vi "data normalization.vi"() -> ()   [LabVIEW 2025]
panel:
  out "spreadsheet string":string
  out "1D array size":i32
  out "array 2":dbl[](array[numeric])
  out "# of columns":i32
  out "x = y?":bool
  in  "1D worksheet for data processing":string="2.000E+0\t-9.081E-1\t\n2.000E+0\t-9.082E-1\t\n2.000E+0\t-9.083E-1\t\n2.000E+0\t-9.081E-1\t\n2.000E+0\t-9.083E-1\t\n1.750E+0\t-9.075E-1\t\n1.750E+0\t-9.076E-1\t\n1.750E+0\t-9.073E-1\t\n1.750E+0\t-9.075E-1\t\n1.750E+0\t-9.075E-1\t\n1.500E+0\t-9.067E-1\t\n1.500E+0\t-9.068E-1\t\n1.500E+0\t-9.067E-1\t\n1.500E+0\t-9.067E-1\t\n1.500E+0\t-9.067E-1\t\n1.250E+0\t-9.057E-1\t\n1.250E+0\t-9.060E-1\t\n1.250E+0\t-9.059E-1\t\n1.250E+0\t-9.059E-1\t\n1.250E+0\t-9.057E-1\t\n1.000E+0\t-9.109E-1\t\n1.000E+0\t-9.109E-1\t\n1.000E+0\t-9.109E-1\t\n1.000E+0\t-9.108E-1\t\n1.000E+0\t-9.109E-1\t\n7.500E-1\t-9.041E-1\t\n7.500E-1\t-9.042E-1\t\n7.500E-1\t-9.042E-1\t\n7.500E-1\t-9.042E-1\t\n7.500E-1\t-9.042E-1\t\n5.000E-1\t-9.032E-1\t\n5.000E-1\t-9.031E-1\t\n2.000E+0\t-9.086E-1\t\n1.890E+0\t-9.080E-1\t\n1.780E+0\t-9.078E-1\t\n1.670E+0\t-9.074E-1\t\n1.560E+0\t-9.070E-1\t\n1.450E+0\t-9.068E-1\t\n1.340E+0\t-9.121E-1\t\n1.230E+0\t-9.058E-1\t\n1.120E+0\t-9.054E-1\t\n1.010E+0\t-9.111E-1\t\n9.000E-1\t-9.048E-1\t\n7.900E-1\t-9.044E-1\t\n6.800E-1\t-9.038E-1\t\n6.300E-1\t-9.037E-1\t\n5.800E-1\t-9.037E-1\t\n5.300E-1\t-9.033E-1\t\n4.800E-1\t-9.034E-1\t\n4.300E-1\t-9.029E-1\t\n3.800E-1\t-9.029E-1\t\n3.300E-1\t-9.043E-1\t\n2.800E-1\t-9.059E-1\t\n2.300E-1\t-9.135E-1\t\n1.800E-1\t-9.091E-1\t\n1.300E-1\t-9.108E-1\t\n8.000E-2\t-9.123E-1\t\n0.000E+0\t-9.211E-1\t"
  in  "2D Data worksheet":string="2.000E+0\t-9.081E-1\t\n2.000E+0\t-9.082E-1\t\n2.000E+0\t-9.083E-1\t\n2.000E+0\t-9.081E-1\t\n2.000E+0\t-9.083E-1\t\n1.750E+0\t-9.075E-1\t\n1.750E+0\t-9.076E-1\t\n1.750E+0\t-9.073E-1\t\n1.750E+0\t-9.075E-1\t\n1.750E+0\t-9.075E-1\t\n1.500E+0\t-9.067E-1\t\n1.500E+0\t-9.068E-1\t\n1.500E+0\t-9.067E-1\t\n1.500E+0\t-9.067E-1\t\n1.500E+0\t-9.067E-1\t\n1.250E+0\t-9.057E-1\t\n1.250E+0\t-9.060E-1\t\n1.250E+0\t-9.059E-1\t\n1.250E+0\t-9.059E-1\t\n1.250E+0\t-9.057E-1\t\n1.000E+0\t-9.109E-1\t\n1.000E+0\t-9.109E-1\t\n1.000E+0\t-9.109E-1\t\n1.000E+0\t-9.108E-1\t\n1.000E+0\t-9.109E-1\t\n7.500E-1\t-9.041E-1\t\n7.500E-1\t-9.042E-1\t\n7.500E-1\t-9.042E-1\t\n7.500E-1\t-9.042E-1\t\n7.500E-1\t-9.042E-1\t\n5.000E-1\t-9.032E-1\t\n5.000E-1\t-9.031E-1\t\n2.000E+0\t-9.086E-1\t\n1.890E+0\t-9.080E-1\t\n1.780E+0\t-9.078E-1\t\n1.670E+0\t-9.074E-1\t\n1.560E+0\t-9.070E-1\t\n1.450E+0\t-9.068E-1\t\n1.340E+0\t-9.121E-1\t\n1.230E+0\t-9.058E-1\t\n1.120E+0\t-9.054E-1\t\n1.010E+0\t-9.111E-1\t\n9.000E-1\t-9.048E-1\t\n7.900E-1\t-9.044E-1\t\n6.800E-1\t-9.038E-1\t\n6.300E-1\t-9.037E-1\t\n5.800E-1\t-9.037E-1\t\n5.300E-1\t-9.033E-1\t\n4.800E-1\t-9.034E-1\t\n4.300E-1\t-9.029E-1\t\n3.800E-1\t-9.029E-1\t\n3.300E-1\t-9.043E-1\t\n2.800E-1\t-9.059E-1\t\n2.300E-1\t-9.135E-1\t\n1.800E-1\t-9.091E-1\t\n1.300E-1\t-9.108E-1\t\n8.000E-2\t-9.123E-1\t\n0.000E+0\t-9.211E-1\t"
  # "Modify the diagram inside the For Loop"
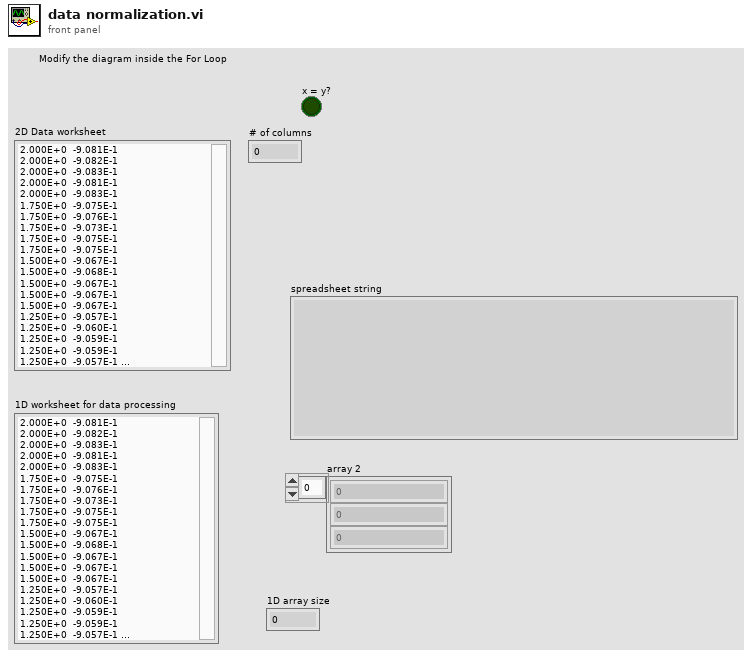
[diagram p1: front panel]
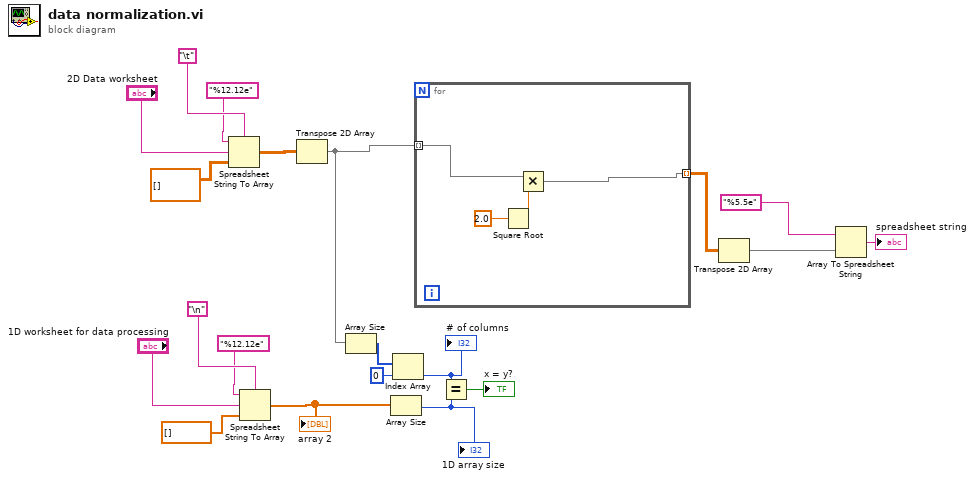
[diagram p0: block diagram]
diagram:
  n1 = Spreadsheet String To Array(delimiter (Tab)="\t", format string="%12.12e", spreadsheet string="2D Data worksheet", array type (2D Dbl)=dbl[][] []) -> (array=w16:dbl[][])
  n2 = Spreadsheet String To Array(delimiter (Tab)="\n", format string="%12.12e", spreadsheet string="1D worksheet for data processing", array type (2D Dbl)=dbl[] []) -> (array=w11:dbl[])
  "array 2" <- w11
  n3 = Transpose 2D Array(2D array=w16) -> (transposed array=w9:dbl[][])
  n4 = Array Size(array=w9) -> (size(s)=w8:i32[])
  n5 = Array Size(array=w11) -> (size(s)=w10:i32)
  "1D array size" <- w10
  n6 = Index Array(array=w8, index=0) -> (element=w6:i32)
  "# of columns" <- w6
  n7 = for {
    tunnel: w9 -> [w24] mode=indexing
    tunnel: [w21] -> w3 mode=indexing
    n8 = Square Root(x=2.0) -> (sqrt(x)=w22:dbl)
    n9 = Multiply(x=w24, y=w22) -> (x*y=w21:dbl[])
  }
  n10 = Equal?(x=w6, y=w10) -> (x = y?=→"x = y?":bool)
  n11 = Transpose 2D Array(2D array=w3) -> (transposed array=w1:dbl[][])
  n12 = Array To Spreadsheet String(array=w1, 3:"%5.5e" ("format string")) -> (spreadsheet string=→"spreadsheet string":string)  [unwired: 1 out]
